vi "subSaveImage_v2.vi"(7 "File name":path=path "" caption="start path", 8 "Camera error in":errorcluster caption="File error", 9 "Exposure (msec)":dbl=100.0 min=1.0 max=5000.0 step=1.0) -> (0 "Camera error out":errorcluster, 2 "Image Data":dbl[][](array[numeric]))   [LabVIEW 2012]
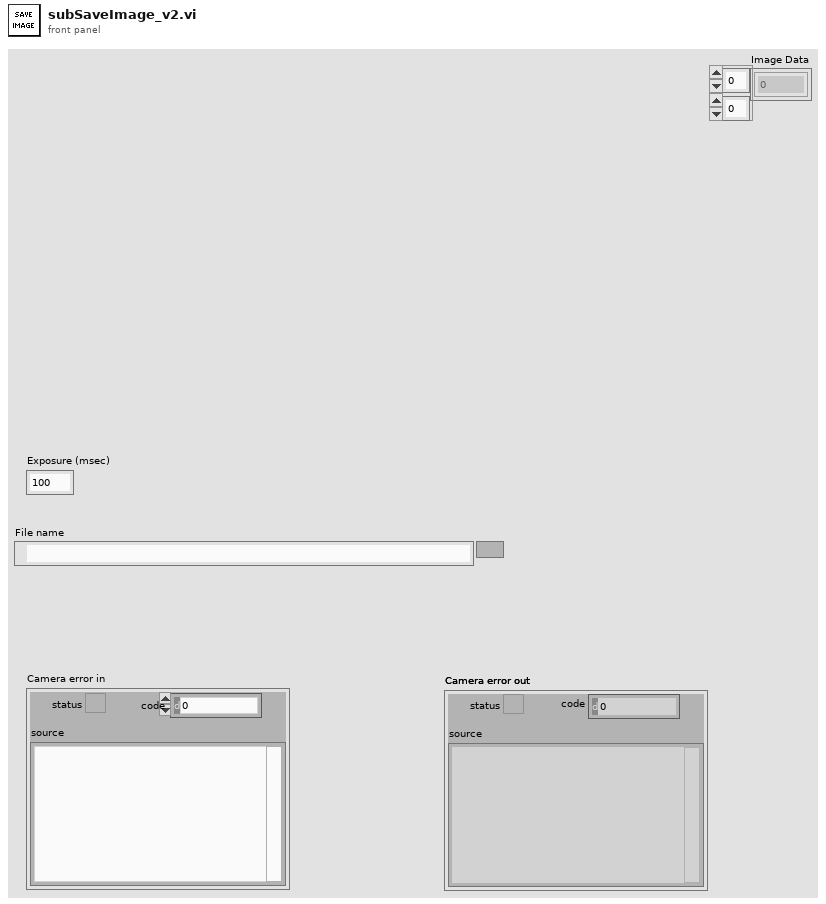
[diagram p1: front panel]
types:
  T1 = cluster{"width":u32, "height":u32, "datatype":u32}
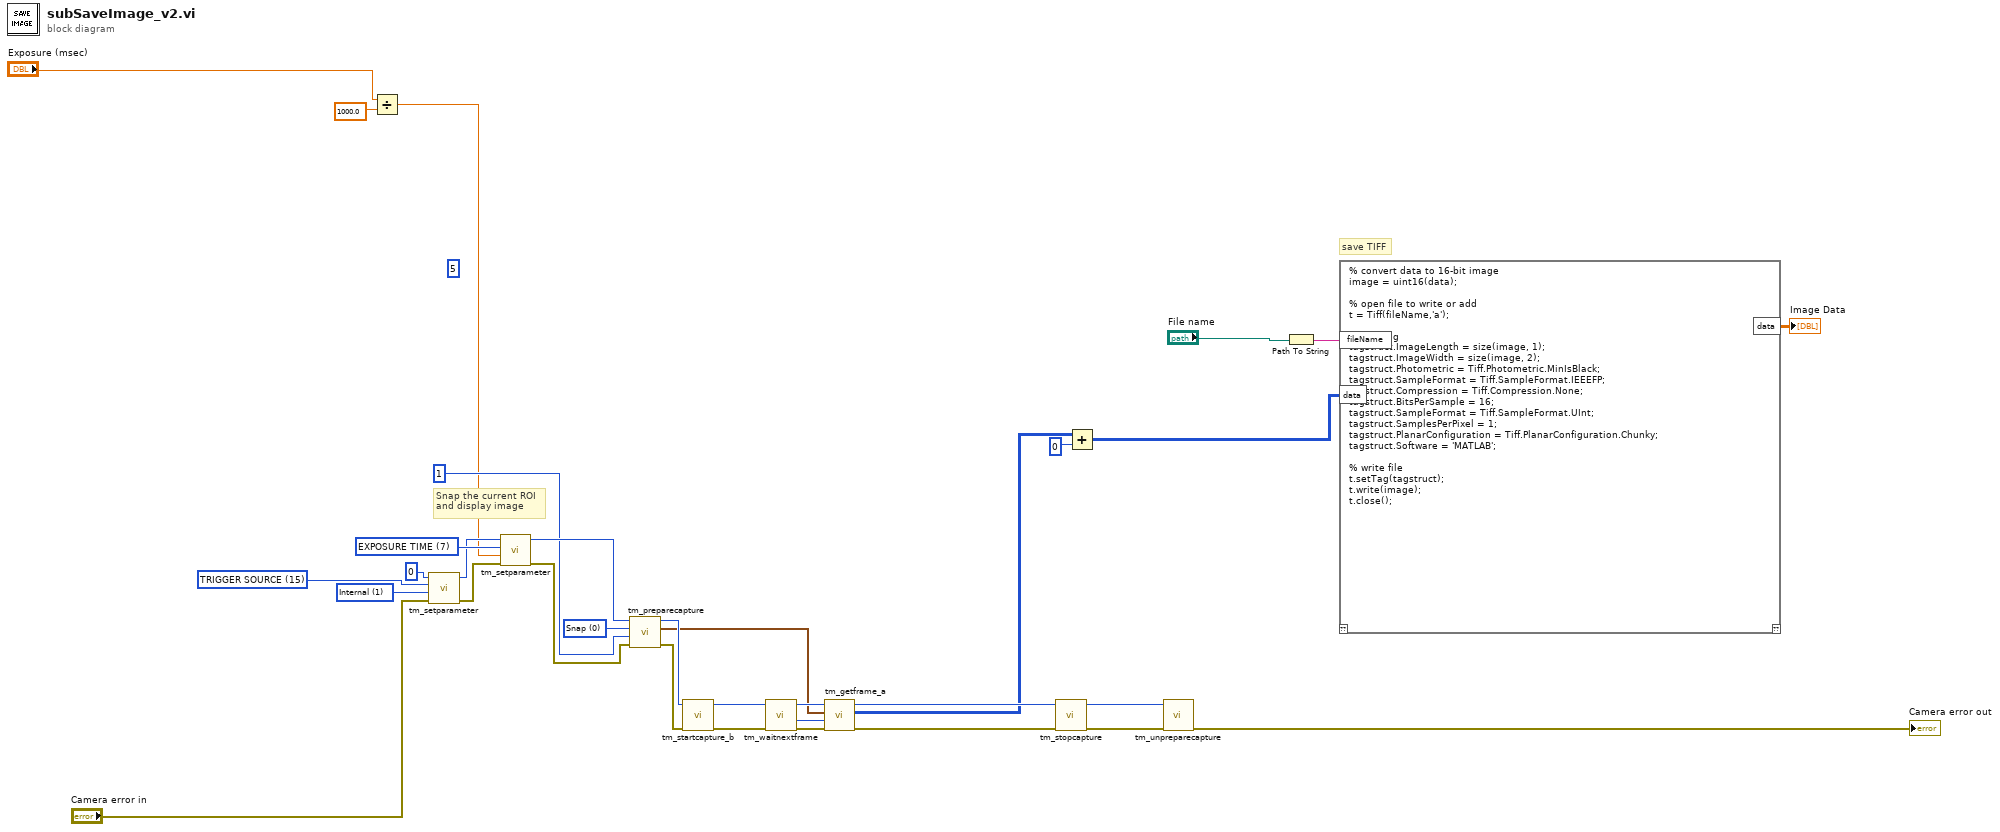
[diagram p0: block diagram]
diagram:
  (unwired) 5
  w24 = 0 items=["Snap", "Sequence"] ("Capture mode")
  w30 = 1 items=["Internal"=1, "External"=2, "Software"=3] ("Trigger Source")
  w29 = 7 items=["BINNING"=1, "BITS PER CHANNEL"=2, "ACTIVE VIEW INDEX"=3, "CCD MODE"=4, "SENSOR MODE"=5, "READOUT MODE"=6, "EXPOSURE TIME"=7, "CONTRAST GAIN"=8, "CONTRAST OFFSET"=9, "LIGHT MODE"=10, "SENSITIVITY"=11, "WHITE BALANCE"=12, "PHOTON IMAGING MODE"=13, "HIGH DYNAMIC RANGE MODE"=14, "TRIGGER SOURCE"=15, "TRIGGER ACTIVE"=16, "TRIGGER MODE"=17, "TRIGGER POLARITY"=18, "TRIGGER GLOBAL EXPOSURE"=19, "FIRST TRIGGER BEHAVIOR"=20, "TRIGGER TIMES"=21, "OUTPUT TRIGGER POLARITY"=22, "OUTPUT TRIGGER DELAY"=23, "OUTPUT TRIGGER PERIOD"=24, "TEMPERATURE"=25, "TEMPERATURE TARGET"=26, "SENSOR COOLER FAN"=27, "MECHANICAL SHUTTER"=28, "BACK FOCUS POSITION"=29, "FRAMEBUNDLE MODE"=30, "FRAMEBUNDLE NUMBER"=31, "LINEBUNDLE HEIGHT"=32, "TRIGGER CONNECTOR"=33, "IMAGE PIXEL TYPE"=34] ("Parameter")
  w31 = 15 items=["BINNING"=1, "BITS PER CHANNEL"=2, "ACTIVE VIEW INDEX"=3, "CCD MODE"=4, "SENSOR MODE"=5, "READOUT MODE"=6, "EXPOSURE TIME"=7, "CONTRAST GAIN"=8, "CONTRAST OFFSET"=9, "LIGHT MODE"=10, "SENSITIVITY"=11, "WHITE BALANCE"=12, "PHOTON IMAGING MODE"=13, "HIGH DYNAMIC RANGE MODE"=14, "TRIGGER SOURCE"=15, "TRIGGER ACTIVE"=16, "TRIGGER MODE"=17, "TRIGGER POLARITY"=18, "TRIGGER GLOBAL EXPOSURE"=19, "FIRST TRIGGER BEHAVIOR"=20, "TRIGGER TIMES"=21, "OUTPUT TRIGGER POLARITY"=22, "OUTPUT TRIGGER DELAY"=23, "OUTPUT TRIGGER PERIOD"=24, "TEMPERATURE"=25, "TEMPERATURE TARGET"=26, "SENSOR COOLER FAN"=27, "MECHANICAL SHUTTER"=28, "BACK FOCUS POSITION"=29, "FRAMEBUNDLE MODE"=30, "FRAMEBUNDLE NUMBER"=31, "LINEBUNDLE HEIGHT"=32, "TRIGGER CONNECTOR"=33, "IMAGE PIXEL TYPE"=34] ("Parameter")
  # "save TIFF"
  # "Snap the current ROI\nand display image"
  n1 = Divide(x="Exposure (msec)", y=1000.0) -> (x/y=w7:dbl)
  n2 = call <userlib>:"tm_setparameter.vi"("error in (no error)"="Camera error in", "Value in"=w30, "Parameter"=w31, "Handle in"=u32 0) -> ("error out"=w28:errorcluster, "Handle out"=w26:u32)  [unwired: 6 in]
  n3 = call <userlib>:"tm_setparameter.vi"("error in (no error)"=w28, "Value in"=w7, "Parameter"=w29, "Handle in"=w26) -> ("error out"=w32:errorcluster, "Handle out"=w33:u32)  [unwired: 6 in]
  n4 = call <userlib>:"tm_preparecapture.vi"("error in (no error)"=w32, "Frames"=1, "Capture mode"=w24, "Handle in"=w33) -> ("error out"=w23:errorcluster, "Buffer"=w16:T1, "Handle out"=w22:u32)  [unwired: 4 in, 1 out]
  n5 = call <userlib>:"tm_startcapture_b.vi"("error in (no error)"=w23, "Handle in"=w22) -> ("error out"=w21:errorcluster, "Handle out"=w20:u32)  [unwired: 8 in]
  n6 = call <userlib>:"tm_waitnextframe.vi"("error in (no error)"=w21, "Handle in"=w20) -> ("error out"=w19:errorcluster, "Frame Count"=w18:i32, "Handle out"=w17:u32)  [unwired: 6 in, 1 out]
  n7 = call <userlib>:"tm_getframe_a.vi"("error in (no error)"=w19, "Frame Index"=w18, "Buffer"=w16, "Handle in"=w17) -> ("error out"=w15:errorcluster, "Data 16"=w11:u16[][], "Handle out"=w14:u32)  [unwired: 4 in, 1 out]
  n8 = call <userlib>:"tm_stopcapture.vi"("error in (no error)"=w15, "Handle in"=w14) -> ("error out"=w13:errorcluster, "Handle out"=w12:u32)  [unwired: 8 in]
  n9 = Add(x=w11, y=0) -> (x+y=w10:i32[][])
  n10 = call <userlib>:"tm_unpreparecapture.vi"("error in (no error)"=w13, "Handle in"=w12) -> ("error out"=→"Camera error out":errorcluster)  [unwired: 8 in, 1 out]
  n11 = Path To String(path="File name") -> (string=w4:string)
  n12 = script code="% convert data to 16-bit image\nimage = uint16(data);\n\n% open file to write or add\nt = Tiff(fileName,'a');\n\n% edit tag\ntagstruct.ImageLength = size(image, 1);\ntagstruct.ImageWidth = size(image, 2);\ntagstruct.Photometric = Tiff.Photometric.MinIsBlack;\ntagstruct.SampleFormat = Tiff.SampleFormat.IEEEFP;\ntagstruct.Compression = Tiff.Compression.None;\ntagstruct.BitsPerSample = 16;\ntagstruct.SampleFormat = Tiff.SampleFormat.UInt;\ntagstruct.SamplesPerPixel = 1;\ntagstruct.PlanarConfiguration = Tiff.PlanarConfiguration.Chunky;\ntagstruct.Software = 'MATLAB';\n\n% write file\nt.setTag(tagstruct);\nt.write(image);\nt.close();"("fileName"=w4, "data"=w10) -> ("data"=→"Image Data":dbl[][])  [unwired: 1 in, 1 out]
